vi "CheckValues_config_estacionXML.vi"(8 "error in (no error)":errorcluster, 11 "Coordenadas_estacion":T1) -> (0 "error out":errorcluster, 3 "XML NULL?":bool)   [LabVIEW 2019]
uses:
  LVPROJ_CONFIG_ESTACION/Type_defs/Coordenadas_estacion.ctl
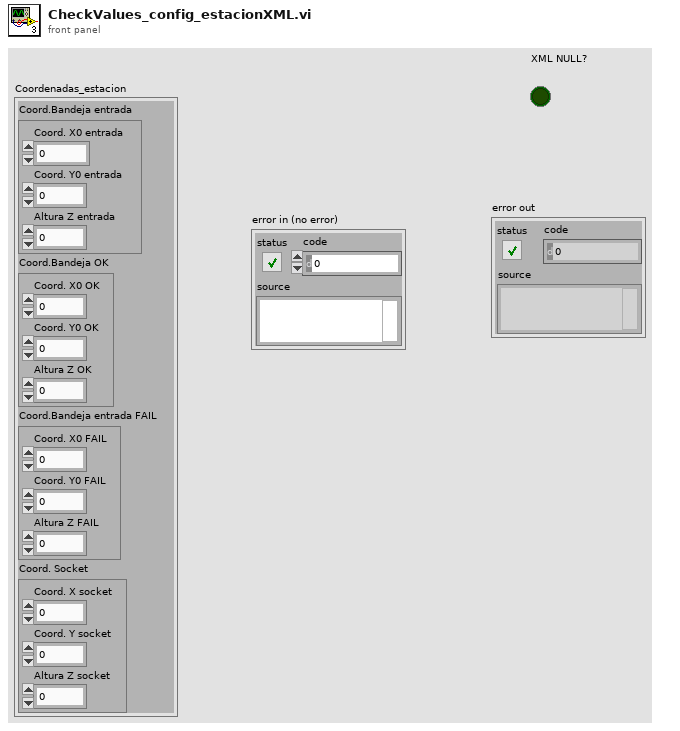
[diagram p1: front panel]
types:
  T1 = typedef "Coordenadas_estacion.ctl" = cluster{"Coord.Bandeja entrada":cluster{"Coord. X0 entrada":u32, "Coord. Y0 entrada ":u32, "Altura Z entrada":u32}, "Coord.Bandeja OK":cluster{"Coord. X0 OK":u32, "Coord. Y0 OK":u32, "Altura Z OK":u32}, "Coord.Bandeja entrada FAIL":cluster{"Coord. X0 FAIL":u32, "Coord. Y0 FAIL":u32, "Altura Z FAIL":u32}, "Coord. Socket":cluster{"Coord. X socket":u32, "Coord. Y socket":u32, "Altura Z socket":u32}}
  T2 = cluster{"Coord.Bandeja entrada":cluster{"Coord. X0 entrada":bool, "Coord. Y0 entrada ":bool, "Altura Z entrada":bool}, "Coord.Bandeja OK":cluster{"Coord. X0 OK":bool, "Coord. Y0 OK":bool, "Altura Z OK":bool}, "Coord.Bandeja entrada FAIL":cluster{"Coord. X0 FAIL":bool, "Coord. Y0 FAIL":bool, "Altura Z FAIL":bool}, "Coord. Socket":cluster{"Coord. X socket":bool, "Coord. Y socket":bool, "Altura Z socket":bool}}
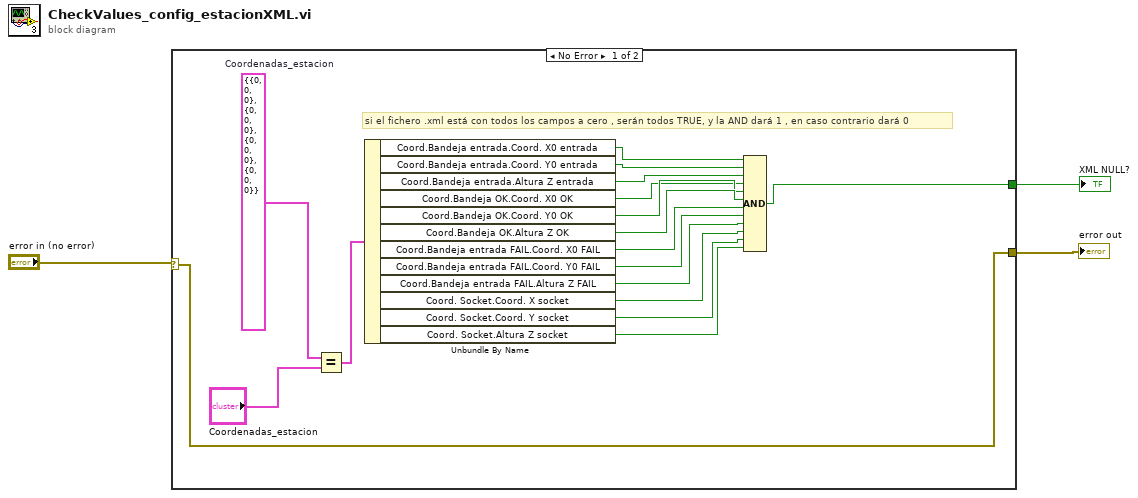
[diagram p0: block diagram]
diagram:
  n1 = case shown="No Error" "error in (no error)" {
    selector: "error in (no error)" -> [w5 w21]
    tunnel: [w5 w21] -> w2
    tunnel: [w4 _] -> w1
    frame No Error {
      w6 = T1 {"Coord.Bandeja entrada"={"Coord. X0 entrada"=0, "Coord. Y0 entrada "=0, "Altura Z entrada"=0}, "Coord.Bandeja OK"={"Coord. X0 OK"=0, "Coord. Y0 OK"=0, "Altura Z OK"=0}, "Coord.Bandeja entrada FAIL"={"Coord. X0 FAIL"=0, "Coord. Y0 FAIL"=0, "Altura Z FAIL"=0}, "Coord. Socket"={"Coord. X socket"=0, "Coord. Y socket"=0, "Altura Z socket"=0}}  # Coordenadas_estacion
      # "si el fichero .xml está con todos los campos a cero , serán todos TRUE, y la AND dará 1 , en caso contrario dará 0"
      n2 = Equal?(x=w6, y="Coordenadas_estacion") -> (x = y?=w8:T2)
      n3 = Unbundle By Name(w8) -> ("Coord.Bandeja entrada.Coord. X0 entrada"=w9:bool, "Coord.Bandeja entrada.Coord. Y0 entrada"=w10:bool, "Coord.Bandeja entrada.Altura Z entrada"=w11:bool, "Coord.Bandeja OK.Coord. X0 OK"=w12:bool, "Coord.Bandeja OK.Coord. Y0 OK"=w13:bool, "Coord.Bandeja OK.Altura Z OK"=w14:bool, "Coord.Bandeja entrada FAIL.Coord. X0 FAIL"=w15:bool, "Coord.Bandeja entrada FAIL.Coord. Y0 FAIL"=w16:bool, "Coord.Bandeja entrada FAIL.Altura Z FAIL"=w17:bool, "Coord. Socket.Coord. X socket"=w18:bool, "Coord. Socket.Coord. Y socket"=w19:bool, "Coord. Socket.Altura Z socket"=w20:bool)
      n4 = Compound Arithmetic op=AND(w9, w10, w11, w12, w13, w14, w15, w16, w17, w18, w19, w20) -> (w4:bool)
    }
    frame Error {
    }
  }
  "error out" <- w2
  "XML NULL?" <- w1
